vi "LogData.vi"(8 "error in (no error)":errorcluster, 10 "Start time":u32, 11 "Refmum":refnum<file>) -> (0 "error out":errorcluster, 3 "Byte Stream File out":refnum<file>)   [LabVIEW 2018]
doc: "This VI writes one line of data to the log file. Needs to be put in a loop."
uses:
  LogOperation.ctl
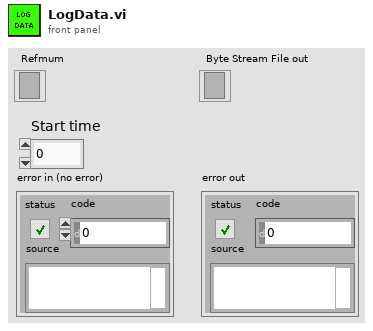
[diagram p1: front panel]
types:
  T1 = typedef "LogOperation.ctl" = enum16{"Set", "Get All", "Get Headers"}
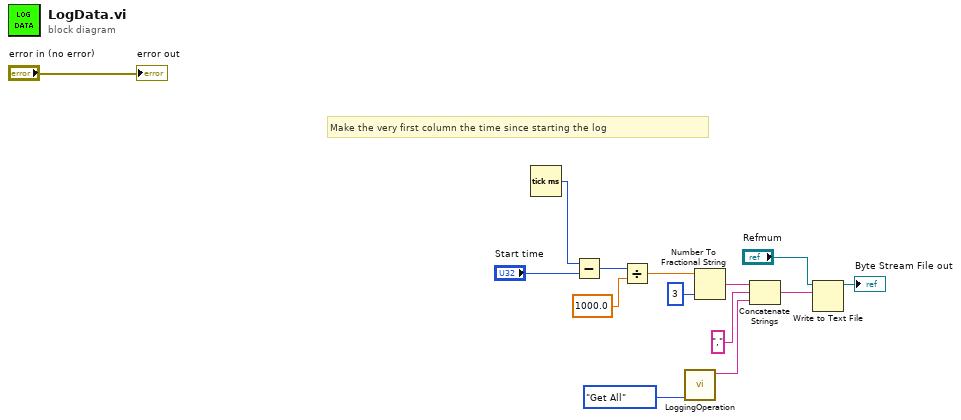
[diagram p0: block diagram]
diagram:
  # "Make the very first column the time since starting the log"
  n1 = Tick Count (ms)() -> (millisecond timer value=w13:u32)
  n2 = Subtract(x=w13, y="Start time") -> (x-y=w11:u32)
  n3 = Divide(x=w11, y=1000.0 ("input 9")) -> (x/y=w6:dbl)
  n4 = call "LoggingOperation.vi"("Operation"=LogOperation."Get All") -> ("Log String"=w2:string)  [unwired: 10 in]
  n5 = Number To Fractional String(number=w6, precision (6)=i16 3) -> (F-format string=w4:string)  [unwired: 2 in]
  n6 = Concatenate Strings(w4, "," ("string"), w2) -> (w1:string)
  n7 = Write to Text File(file (use dialog)="Refmum", text=w1) -> (refnum out=→"Byte Stream File out":refnum<file>)  [unwired: 2 in, 2 out]
  "error out" <- "error in (no error)"
